vi "Main.vi"() -> ()   [LabVIEW 2013]
uses:
  <vilib>/Platform/TimedLoop/XDataNode/timing_clust.ctl
  <vilib>/Platform/TimedLoop/XDataNode/nitl_modes.ctl
  <vilib>/Platform/TimedLoop/XDataNode/wakeup.ctl
  <vilib>/platform/TimedLoop/XDataNode/XDataNode.xnode
  <vilib>/Platform/TimedLoop/XDataNode/XDNodeRunTimeDep.lvlib
panel:
  out "time":timestamp
  in  "ESC":bool
  # "NTP Clock"
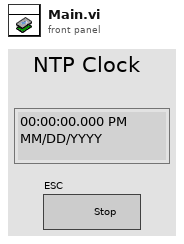
[diagram p1: front panel]
types:
  T1 = typedef "XDNodeRunTimeDep.lvlib/timing_clust.ctl" = cluster{"Expected End [f-1]":u64, "Actual End [f-1]":u64, "Finished Late? [f-1]":bool, "Expected End [i-1]":u64, "Actual End [i-1]":u64, "Finished Late? [i-1]":bool, "Expected Start [i]":u64, "Actual Start [i]":u64, "Expected Start [f]":u64, "Actual Start [f]":u64, "Source Name":string, "Structure Name":string, "Period":i64, "Deadline":i64, "Offset":i64, "Start":i64, "Priority":i32, "Timeout":i32, "Mode":T2, "Wakeup Reason":T3, "Error":errorcluster, "Source Type":string, "Secondary Source Type":string, "Global End Time":u64, "Global Start Time":u64, "Frame Duration":u64, "Iteration Duration":u64, "Assigned CPU":i32, "I/O Scan Engine Mode":u32}
  T2 = typedef "XDNodeRunTimeDep.lvlib/nitl_modes.ctl" = enum32{"No Change", "Process missed periods, maintain original phase", "Discard missed periods, maintain original phase", "Process missed periods, ignore original phase", "Discard missed periods, ignore original phase"}
  T3 = typedef "XDNodeRunTimeDep.lvlib/wakeup.ctl" = enum32{"Normal", "Aborted", "Asynchronous wakeup", "Timing source error", "Timed loop error", "Timeout"}
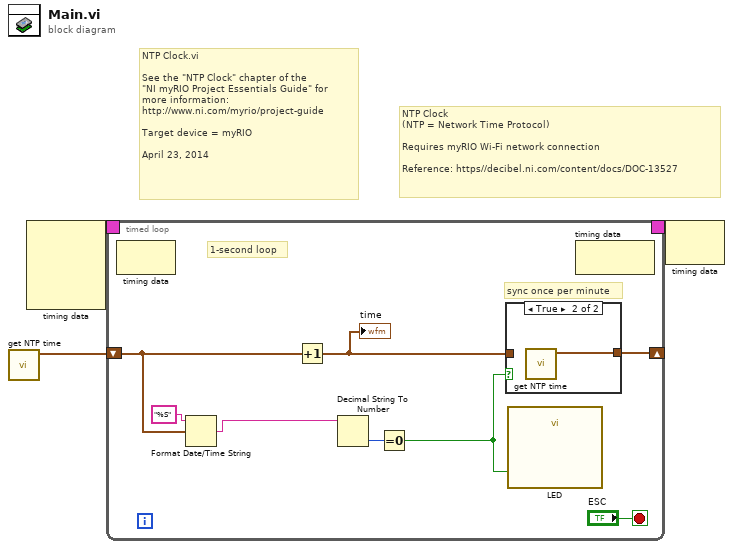
[diagram p0: block diagram]
diagram:
  # "NTP Clock.vi\n\nSee the \"NTP Clock\" chapter of the \n\"NI myRIO Project Essentials Guide\" for\nmore information: \nhttp://www.ni.com/myrio/project-guide\n\nTarget device = myRIO\n\nApril 23, 2014"
  # "NTP Clock\n(NTP = Network Time Protocol)\n\nRequires myRIO Wi-Fi network connection\n\nReference: https//decibel.ni.com/content/docs/DOC-13527"
  n1 = call "get NTP time.vi"() -> ("NTP time"=w1:timestamp)  [unwired: 9 in, 2 out]
  n2 = node-c288() -> (w3:T1)  [unwired: 4 in]
  n3 = timed-loop {
    timing: w3 -> [_]
    timing-out: [_] -> w2
    shift-right: [w10] -> _
    shift-left: w1 -> [w6]
    stop <- "ESC" stop-if-true
    # "1-second loop"
    # "sync once per minute"
    n4 = node-c288() -> ()  [unwired: 1 in, 1 out]
    n5 = Format Date/Time String(time format string (%c)="%S", seconds (now)=w6) -> (date/time string=w5:string)  [unwired: 1 in]
    n6 = Increment(x=w6) -> (x+1=w9:timestamp)
    "time" <- w9
    n7 = Decimal String To Number(string=w5) -> (number=w4:i32)  [unwired: 2 in, 1 out]
    n8 = Equal To 0?(x=w4) -> (x = 0?=w8:bool)
    n9 = case shown="True" w8 {
      tunnel: [w12 w13] -> w10
      tunnel: w9 -> [w12 _]
      frame False {
      }
      frame True {
        n10 = call "get NTP time.vi"() -> ("NTP time"=w13:timestamp)  [unwired: 9 in, 2 out]
      }
    }
    n11 = call "LED"("LED0"=w8) -> ()  [unwired: 26 in, 1 out]
    n12 = node-c288() -> ()  [unwired: 1 in, 1 out]
  }
  n13 = node-c288(w2) -> ()  [unwired: 1 out]
